vi "Get image date.vi"(8 "error in (no error)":errorcluster, 11 "CCDCamera in":refnum<class "iKon-L.lvclass">) -> (0 "error out":errorcluster, 3 "CCDCamera out":refnum<class "iKon-L.lvclass">)   [LabVIEW 2018, in "iKon-L.lvclass"]
doc: "Get the time stamp (in UTC) at the begining of the exposure"
uses:
  iKon-L.lvclass
  C:/Users/Denis/Desktop/S4ACS/S4ACS/Sim_CCD/Sim_CCD.lvclass
  <vilib>/Utility/miscctls.llb/LVDateTimeRec.ctl
  Sim_CCD/Sim_CCD.lvclass
panel:
  in  "date time rec":T1
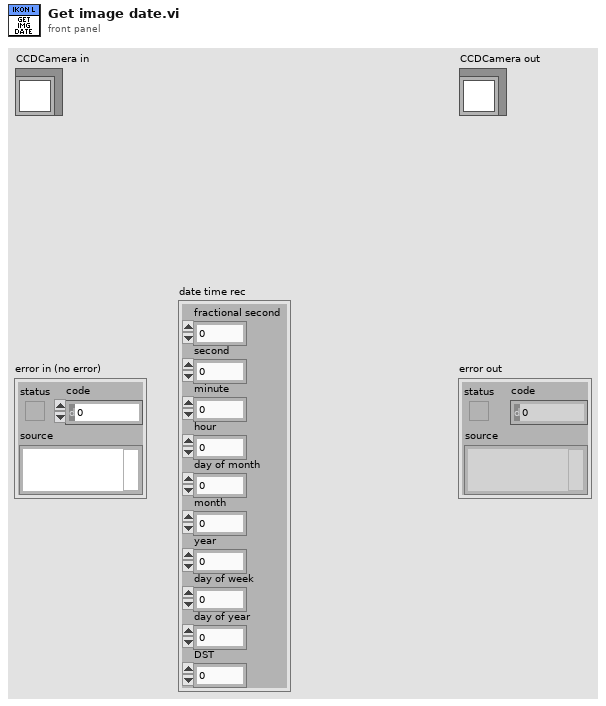
[diagram p1: front panel]
types:
  T1 = typedef "LVDateTimeRec.ctl" = cluster{"fractional second":dbl, "second":i32, "minute":i32, "hour":i32, "day of month":i32, "month":i32, "year":i32, "day of week":i32, "day of year":i32, "DST":i32}
  T2 = cluster{"Time Acq Started":u32, "Image delay":u64, "Last update - CCD config":timestamp, "SYSTEMTIME":T1, "Readout time":dbl, "Time acq finished":u32, "effective exptime":dbl}
  T3 = cluster{"FRAMES_DONE":u16, "CCD_STATUS":string, "CURRENT_TEMPERATURE":i16, "TEMPERATURE_STATUS":string, "FRAME_EXPOSURE_TIME":dbl, "SERIAL_NUMBER":u16, "ACQUIRING":bool, "POWER":bool, "ACS MODE":bool}
  T4 = typedef "SYSTEMTIME structure typedef.ctl" = cluster{"Year":u16, "Month":u16, "DayOfWeek":u16, "Date":u16, "Hour":u16, "Minute":u16, "Second":u16, "Milliseconds":u16}
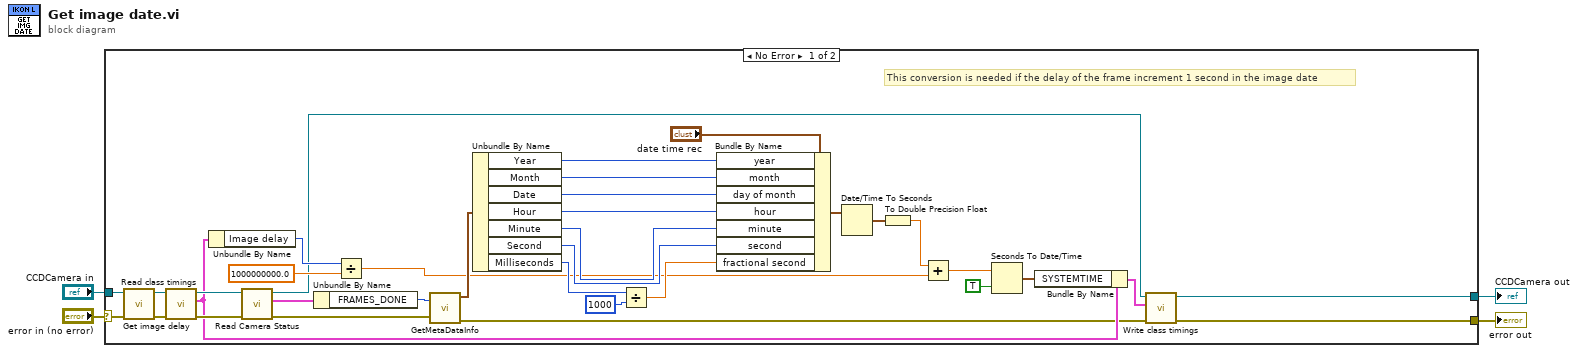
[diagram p0: block diagram]
diagram:
  n1 = case shown="No Error" "error in (no error)" {
    selector: "error in (no error)" -> [w20 w40]
    tunnel: [w9 w40] -> w3
    tunnel: "CCDCamera in" -> [w19 w41]
    tunnel: [w10 w41] -> w1
    frame No Error {
      # "This conversion is needed if the delay of the frame increment 1 second in the image date"
      n2 = call-dynamic "Get image delay.vi"("error in (no error)"=w20, "CCDCamera in"=w19) -> ("error out"=w16:errorcluster, "CCDCamera out"=w15:refnum<class "iKon-L.lvclass">)  [unwired: 8 in]
      n3 = call "Read class timings.vi"("error in (no error)"=w16, "Simulated Camera in"=w15) -> ("error out"=w12:errorcluster, "class timings"=w8:T2, "Simulated Camera out"=w13:refnum<class "iKon-L.lvclass">)  [unwired: 7 in]
      n4 = Unbundle By Name(w8) -> ("Image delay"=w14:u64)
      n5 = call "Read Camera Status.vi"("error in (no error)"=w12, "CCDCamera in"=w13) -> ("error out"=w38:errorcluster, "camera status"=w39:T3, "CCDCamera out"=w11:refnum<class "iKon-L.lvclass">)  [unwired: 7 in]
      n6 = Unbundle By Name(w39) -> ("FRAMES_DONE"=w21:u16)
      n7 = Divide(x=w14, y=1000000000.0) -> (x/y=w17:dbl)
      n8 = call <userlib>:"GetMetaDataInfo.vi"("index"=w21, "error in (no error)"=w38) -> ("SYSTEMTIME"=w23:T4, "error out"=w6:errorcluster)  [unwired: 2 out]
      n9 = Unbundle By Name(w23) -> ("Year"=w30:u16, "Month"=w29:u16, "Date"=w28:u16, "Hour"=w27:u16, "Minute"=w26:u16, "Second"=w25:u16, "Milliseconds"=w32:u16)
      n10 = Divide(x=w32, y=1000) -> (x/y=w24:dbl)
      n11 = Bundle By Name(cluster="date time rec", "year"=w30, "month"=w29, "day of month"=w28, "hour"=w27, "minute"=w26, "second"=w25, "fractional second"=w24) -> (w36:T1)
      n12 = Date/Time To Seconds(2:w36) -> (0:w35:timestamp)  [unwired: 1 in]
      n13 = To Double Precision Float(number=w35) -> (double precision float=w34:dbl)
      n14 = Add(x=w34, y=w17) -> (x+y=w33:dbl)
      n15 = Seconds To Date/Time(time stamp (now)=w33, to UTC (F)=TRUE) -> (date time rec=w5:T1)
      n16 = Bundle By Name(cluster=w8, "SYSTEMTIME"=w5) -> (w7:T2)
      n17 = call "Write class timings.vi"("error in (no error)"=w6, "class timings"=w7, "Simulated Camera in"=w11) -> ("error out"=w9:errorcluster, "Simulated Camera out"=w10:refnum<class "iKon-L.lvclass">)  [unwired: 7 in]
    }
    frame Error {
    }
  }
  "error out" <- w3
  "CCDCamera out" <- w1
